vi "Get Compatible HWplugins LUT.vi"(8 "error in (no error)":errorcluster, 10 "Function Name":string, 11 "Controller in":refnum<class "Controller.lvclass">) -> (0 "error out":errorcluster, 2 "HWplugin List LUT (HWType -> Array of HWplugin Objs)":variant, 3 "Controller out":refnum<class "Controller.lvclass">)   [LabVIEW 2016, in "Controller Actor.lvlib" / "Controller.lvclass"]
uses:
  <userlib>/Common Components/Controller/Controller.lvclass
  <userlib>/Common Components/Controller/Controller.lvclass/Controller.ctl
  <userlib>/Common Components/Hardware/Abstract Hardware/Hardware.lvclass
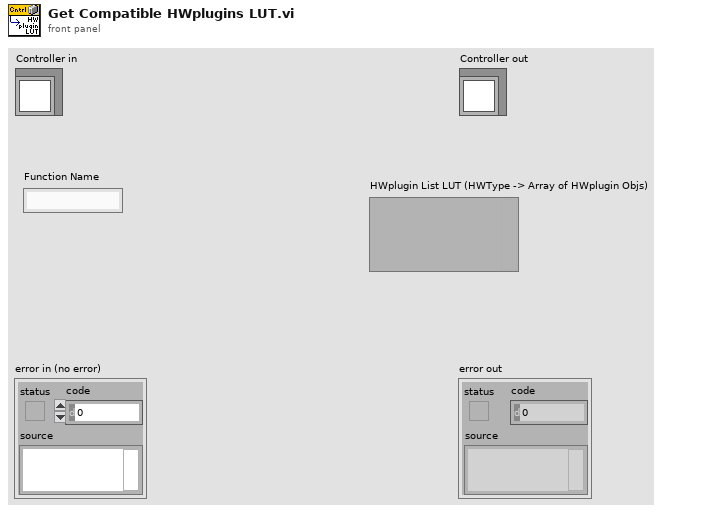
[diagram p1: front panel]
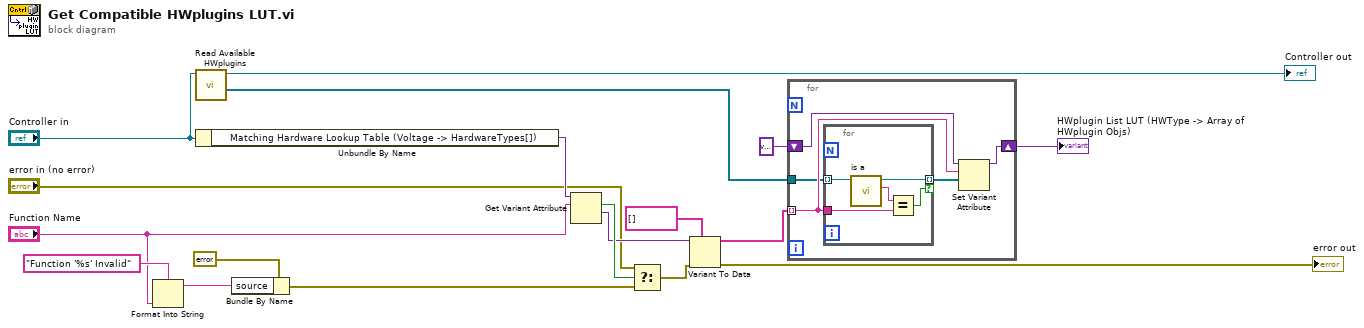
[diagram p0: block diagram]
diagram:
  n1 = Format Into String(format string="Function '%s' Invalid" ("source"), "Function Name") -> (resulting string=w15:string)  [unwired: 2 in, 1 out]
  n2 = call <userlib>:"Read Available HWplugins.vi"("Controller in"="Controller in") -> ("Array of HWplugin Objs"=w5:refnum<class "Hardware.lvclass">[], "Controller out"=→"Controller out":refnum<class "Controller.lvclass">)  [unwired: 7 in, 2 out]
  n3 = Unbundle By Name("Controller in") -> ("Matching Hardware Lookup Table (Voltage -> HardwareTypes[])"=w17:variant)
  n4 = Bundle By Name(cluster=errorcluster {"status"=TRUE, "code"=5559, "source"="Function '%s' Invalid"} ("error constant"), "source"=w15) -> (w13:errorcluster)
  n5 = Get Variant Attribute(Variant=w17, name="Function Name") -> (found=w11:bool, value=w10:variant)  [unwired: 2 in, 2 out]
  n6 = Select(t="error in (no error)", s=w11, f=w13) -> (s? t:f=w3:errorcluster)
  n7 = Variant To Data(error in=w3, type=string[] [], Variant=w10) -> (data=w8:string[], error out=→"error out":errorcluster)
  n8 = for {
    tunnel: w8 -> [w21] mode=indexing
    shift-right: [w22] -> w4
    shift-left: variant -> [w23]
    tunnel: w5 -> [w20]
    n9 = for {
      tunnel: w21 -> [w25]
      tunnel: w20 -> [w28] mode=indexing
      tunnel: [w26] -> w19 mode=indexing if=w27
      n10 = call-dynamic "is a.vi"("Hardware in"=w28) -> ("is a"=w24:string, "Hardware out"=w26:refnum<class "Hardware.lvclass">)  [unwired: 8 in, 1 out]
      n11 = Equal?(x=w24, y=w25) -> (x = y?=w27:bool)
    }
    n12 = Set Variant Attribute(Variant=w23, name=w21, value=w19) -> (Variant out=w22:variant)  [unwired: 1 in, 2 out]
  }
  "HWplugin List LUT (HWType -> Array of HWplugin Objs)" <- w4
